vi "CurrentInput.vi"(8 "Mode":u16(ring) items=["Log w/ Exp Z", "Log w/ Lin Z"], 9 "Maximum (pA)":dbl=9000.0, 10 "Current (pA)":dbl format="%.1f", 11 "Setpoint (pA)":dbl=100.0) -> (2 "Safetip?":bool, 3 "Filtered Current (pA)":dbl format="%.1f")   [LabVIEW 2017]
uses:
  Program Files/National Instruments/LabVIEW 2019/user.lib/HapticSTM/HapticSTM.lvlib
  <vilib>/ptbypt/NI_PtbyPt.lvlib
  <vilib>/Analysis/3filter.llb/Filter Passband Type.ctl
  <vilib>/Analysis/NI_AALBase.lvlib
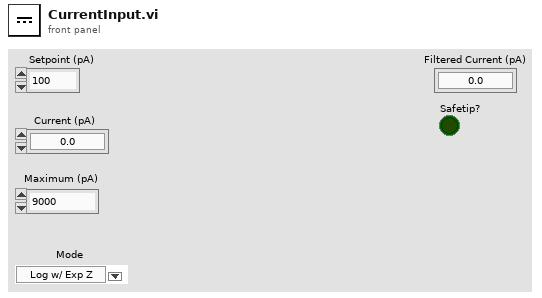
[diagram p1: front panel]
types:
  T1 = typedef "NI_AALBase.lvlib/Filter Passband Type.ctl" = enum32{"Lowpass", "Highpass", "Bandpass", "Bandstop"}
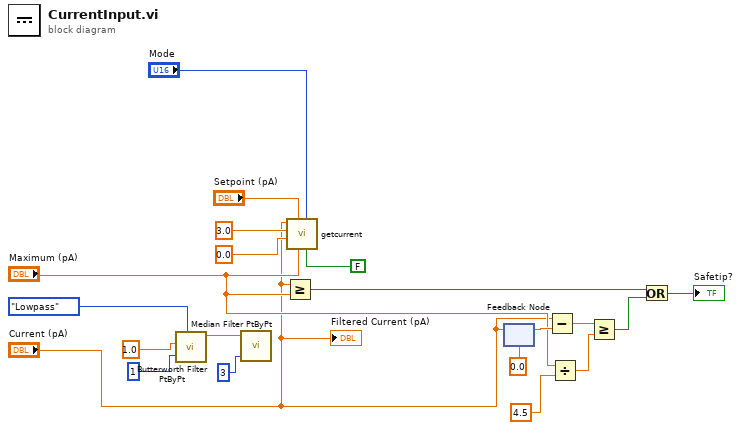
[diagram p0: block diagram]
diagram:
  n1 = call <vilib>:"Butterworth Filter PtByPt.vi"("order"=1, "filter type"=Filter_Passband_Type."Lowpass", "sampling freq: fs"=1.0) -> ("Filtered x"=w15:dbl)  [unwired: 6 in, 1 out]
  n2 = call <vilib>:"Median Filter PtByPt.vi"("rank"=3, "x"=w15) -> ()  [unwired: 2 in, 2 out]
  n3 = Greater Or Equal?(x="Current (pA)", y="Maximum (pA)") -> (x >= y?=w12:bool)
  n4 = call "getcurrent.vi"("afmmode"=FALSE, "forcemode"="Mode", "maxcurrentin"="Maximum (pA)", "setpoint"="Setpoint (pA)", "minforcey"=0.0, "maxforcey"=3.0, "currentin"="Current (pA)") -> ()  [unwired: 5 in]
  n5 = feedback-in #1("Current (pA)") -> ()
  n6 = feedback #1(0.0 ("Current (pA)")) -> (w10:dbl)
  n7 = Subtract(x="Current (pA)", y=w10) -> (x-y=w8:dbl)
  n8 = Divide(x="Maximum (pA)", y=4.5) -> (x/y=w6:dbl)
  n9 = Greater Or Equal?(x=w8, y=w6) -> (x >= y?=w7:bool)
  n10 = Or(x=w12, y=w7) -> (x .or. y?=→"Safetip?":bool)
  "Filtered Current (pA)" <- "Current (pA)"
